vi "SPCReadRates_HH.vi"() -> (0 "error out":errorcluster, 1 "SPC_rates":T1 {"Ch 4" format="%.2e"; "Ch3" format="%.2e"; "Ch2" format="%.2e"; "Ch1" format="%.2e"; "Sync_rate" format="%.2e"})   [LabVIEW 2009]
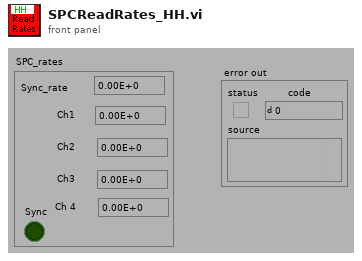
[diagram p1: front panel]
types:
  T1 = cluster{"Sync_rate":sgl, "Ch1":sgl, "Ch2":sgl, "Ch3":sgl, "Ch 4":sgl, "Sync":bool}
  T2 = cluster{"SyncRate":i32, "Rate 1":i32, "Rate 2":i32, "Rate 3":i32, "Rate 4":i32, bool}
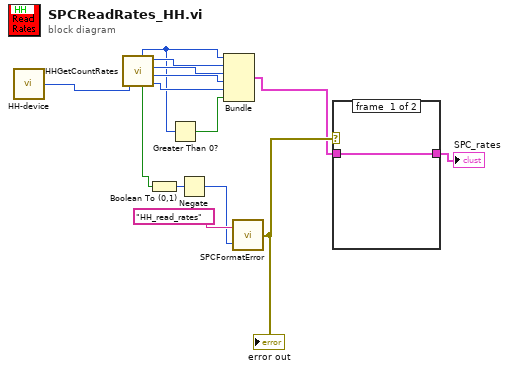
[diagram p0: block diagram]
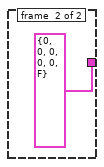
[diagram p2: hidden frame]
diagram:
  n1 = call "HH-device.vi"() -> ("Device (output)"=w11:i32)  [unwired: 2 in]
  n2 = call "HHGetCountRates.vi"("DeviceIndex"=w11) -> ("SyncRate"=w2:i32, "Error"=w10:bool, "Rate 1"=w7:i32, "Rate 2"=w6:i32, "Rate 3"=w5:i32, "Rate 4"=w4:i32)
  n3 = Boolean To (0,1)(Boolean=w10) -> (0, 1=w9:i16)
  n4 = Greater Than 0?(x=w2) -> (x > 0?=w1:bool)
  n5 = Negate(x=w9) -> (-x=w8:i16)
  n6 = Bundle("SyncRate"=w2, "Rate 1"=w7, "Rate 2"=w6, "Rate 3"=w5, "Rate 4"=w4, w1) -> (w3:T2)  [unwired: 1 in]
  n7 = call "SPCFormatError.vi"("Error Code"=w8, "Source"="HH_read_rates") -> ("error out"=w13:errorcluster)
  "error out" <- w13
  n8 = case shown="Error" w13 {
    tunnel: w3 -> [w15 _]
    tunnel: [w15 T2 {"SyncRate"=0, "Rate 1"=0, "Rate 2"=0, "Rate 3"=0, "Rate 4"=0, FALSE}] -> w12
    frame #0 {
    }
    frame #1 {
    }
  }
  "SPC_rates" <- w12
